vi "modbus_Unpuck.vi"(5 "Pair in":T1={"Давление заданное"=0.3, "Давление в системе"=99.99, "Расход заданый"=0.0, "Расход текущий"=0.0, "Объём заданный"=0.0, "Объём текущий"=0.0, "Старт давление"=FALSE, "Старт расход"=FALSE, "Сброс объёма"=FALSE, "plc_control"=FALSE, "lag_control"=FALSE, "mstop_control"=FALSE, "Давление"={"АЦП CH 0"=0.0, "АЦП CH 1"=0.0, "АЦП CH 2"=0.0, "АЦП CH 3"=0.0, "АЦП CH 4"=0.0, "АЦП CH 5"=0.0, "АЦП CH 6"=0.0, "АЦП CH 7"=0.0}, "Modbus"={"Массив чтения"=[], "Массив записи"=[]}} {"Давление"."АЦП CH 7" format="%.3f"; "Давление"."АЦП CH 6" format="%.3f"; "Давление"."АЦП CH 5" format="%.3f"; "Давление"."АЦП CH 4" format="%.3f"; "Давление"."АЦП CH 3" format="%.3f"; "Давление"."АЦП CH 2" format="%.3f"; "Давление"."АЦП CH 1" format="%.3f"; "Давление"."АЦП CH 0" format="%.3f"; "Объём текущий" min=0.0 max=9999.0 step=0.0001 format="%#_5f"; "Объём заданный" min=0.0 max=9999.0 step=0.0001 format="%#_5f"; "Расход текущий" format="%#_5f"; "Расход заданый" min=0.0 max=40.0 step=0.0001 format="%#_5f"; "Давление в системе" format="%.3f"; "Давление заданное" min=0.3 max=100.0 step=0.01 format="%#_5f"}, 6 "Параметры":T3, 7 "Port 2 in":T2={"Давление заданное"=0.3, "Давление MAX заданное"=100.0, "Давление в насосе"=0.0, "Давление в системе"=99.99, "Расход заданый"=0.0, "Расход текущий"=0.0, "Объём заданный"=0.0, "Объём текущий"=0.0, "Позиция насоса %"=0.0, "Ток двигателя"=0.0, "controlMsg"="", "Клапан k_sys"=FALSE, "Клапан k_res"=FALSE, "Клапан k_air"=FALSE, "Вверх"=FALSE, "Домой"=FALSE, "Вниз"=FALSE, "Старт расход"=FALSE, "Старт давление"=FALSE, "Сброс объёма"=FALSE, "Сброс давления Рсис"=FALSE, "Сброс давления Рнас"=FALSE, "Bits"={"plc_control"=FALSE, "lag_control"=FALSE, "mstop_control"=FALSE, "st_home"=FALSE, "error"=FALSE, "mstart"=FALSE, "pair"=FALSE, "startQ"=FALSE, "startP"=FALSE, "volume_Stop"=FALSE}} {"Ток двигателя" format="%#_5f"; "Расход текущий" format="%#_5f"; "Давление в системе" format="%.3f"; "Объём текущий" min=0.0 max=9999.0 step=0.0001 format="%#_5f"; "Объём заданный" min=0.0 max=9999.0 step=0.0001 format="%#_5f"; "Давление MAX заданное" min=0.0 max=100.0 step=0.01 format="%#_5f"; "Давление заданное" min=0.3 max=100.0 step=0.01 format="%#_5f"; "Расход заданый" min=0.0 max=40.0 step=0.0001 format="%#_5f"; "Давление в насосе" format="%.3f"; "Позиция насоса %" scale=0.0..100.0 scale format="%.2f"}, 8 "Error In":errorcluster, 10 "Modbus Read":u16[](array[numeric]), 11 "Port 1 in":T2={"Давление заданное"=0.3, "Давление MAX заданное"=100.0, "Давление в насосе"=0.0, "Давление в системе"=99.99, "Расход заданый"=0.0, "Расход текущий"=0.0, "Объём заданный"=0.0, "Объём текущий"=0.0, "Позиция насоса %"=0.0, "Ток двигателя"=0.0, "controlMsg"="", "Клапан k_sys"=FALSE, "Клапан k_res"=FALSE, "Клапан k_air"=FALSE, "Вверх"=FALSE, "Домой"=FALSE, "Вниз"=FALSE, "Старт расход"=FALSE, "Старт давление"=FALSE, "Сброс объёма"=FALSE, "Сброс давления Рсис"=FALSE, "Сброс давления Рнас"=FALSE, "Bits"={"plc_control"=FALSE, "lag_control"=FALSE, "mstop_control"=FALSE, "st_home"=FALSE, "error"=FALSE, "mstart"=FALSE, "pair"=FALSE, "startQ"=FALSE, "startP"=FALSE, "volume_Stop"=FALSE}} {"Ток двигателя" format="%#_5f"; "Расход текущий" format="%#_5f"; "Давление в системе" format="%.3f"; "Объём текущий" min=0.0 max=9999.0 step=0.0001 format="%#_5f"; "Объём заданный" min=0.0 max=9999.0 step=0.0001 format="%#_5f"; "Давление MAX заданное" min=0.0 max=100.0 step=0.01 format="%#_5f"; "Давление заданное" min=0.3 max=100.0 step=0.01 format="%#_5f"; "Расход заданый" min=0.0 max=40.0 step=0.0001 format="%#_5f"; "Давление в насосе" format="%.3f"; "Позиция насоса %" scale=0.0..100.0 scale format="%.2f"}) -> (0 "Error Out":errorcluster, 1 "Pair out":T1={"Давление заданное"=0.3, "Давление в системе"=99.99, "Расход заданый"=0.0, "Расход текущий"=0.0, "Объём заданный"=0.0, "Объём текущий"=0.0, "Старт давление"=FALSE, "Старт расход"=FALSE, "Сброс объёма"=FALSE, "plc_control"=FALSE, "lag_control"=FALSE, "mstop_control"=FALSE, "Давление"={"АЦП CH 0"=0.0, "АЦП CH 1"=0.0, "АЦП CH 2"=0.0, "АЦП CH 3"=0.0, "АЦП CH 4"=0.0, "АЦП CH 5"=0.0, "АЦП CH 6"=0.0, "АЦП CH 7"=0.0}, "Modbus"={"Массив чтения"=[], "Массив записи"=[]}} {"Давление"."АЦП CH 7" format="%.3f"; "Давление"."АЦП CH 6" format="%.3f"; "Давление"."АЦП CH 5" format="%.3f"; "Давление"."АЦП CH 4" format="%.3f"; "Давление"."АЦП CH 3" format="%.3f"; "Давление"."АЦП CH 2" format="%.3f"; "Давление"."АЦП CH 1" format="%.3f"; "Давление"."АЦП CH 0" format="%.3f"; "Объём текущий" min=0.0 max=9999.0 step=0.0001 format="%#_5f"; "Объём заданный" min=0.0 max=9999.0 step=0.0001 format="%#_5f"; "Расход текущий" format="%#_5f"; "Расход заданый" min=0.0 max=40.0 step=0.0001 format="%#_5f"; "Давление в системе" format="%.3f"; "Давление заданное" min=0.3 max=100.0 step=0.01 format="%#_5f"}, 2 "Port 2 out":T2={"Давление заданное"=0.3, "Давление MAX заданное"=100.0, "Давление в насосе"=0.0, "Давление в системе"=99.99, "Расход заданый"=0.0, "Расход текущий"=0.0, "Объём заданный"=0.0, "Объём текущий"=0.0, "Позиция насоса %"=0.0, "Ток двигателя"=0.0, "controlMsg"="", "Клапан k_sys"=FALSE, "Клапан k_res"=FALSE, "Клапан k_air"=FALSE, "Вверх"=FALSE, "Домой"=FALSE, "Вниз"=FALSE, "Старт расход"=FALSE, "Старт давление"=FALSE, "Сброс объёма"=FALSE, "Сброс давления Рсис"=FALSE, "Сброс давления Рнас"=FALSE, "Bits"={"plc_control"=FALSE, "lag_control"=FALSE, "mstop_control"=FALSE, "st_home"=FALSE, "error"=FALSE, "mstart"=FALSE, "pair"=FALSE, "startQ"=FALSE, "startP"=FALSE, "volume_Stop"=FALSE}} {"Ток двигателя" format="%#_5f"; "Расход текущий" format="%#_5f"; "Давление в системе" format="%.3f"; "Объём текущий" min=0.0 max=9999.0 step=0.0001 format="%#_5f"; "Объём заданный" min=0.0 max=9999.0 step=0.0001 format="%#_5f"; "Давление MAX заданное" min=0.0 max=100.0 step=0.01 format="%#_5f"; "Давление заданное" min=0.3 max=100.0 step=0.01 format="%#_5f"; "Расход заданый" min=0.0 max=40.0 step=0.0001 format="%#_5f"; "Давление в насосе" format="%.3f"; "Позиция насоса %" scale=0.0..100.0 scale format="%.2f"}, 3 "Port 1 out":T2={"Давление заданное"=0.3, "Давление MAX заданное"=100.0, "Давление в насосе"=0.0, "Давление в системе"=99.99, "Расход заданый"=0.0, "Расход текущий"=0.0, "Объём заданный"=0.0, "Объём текущий"=0.0, "Позиция насоса %"=0.0, "Ток двигателя"=0.0, "controlMsg"="", "Клапан k_sys"=FALSE, "Клапан k_res"=FALSE, "Клапан k_air"=FALSE, "Вверх"=FALSE, "Домой"=FALSE, "Вниз"=FALSE, "Старт расход"=FALSE, "Старт давление"=FALSE, "Сброс объёма"=FALSE, "Сброс давления Рсис"=FALSE, "Сброс давления Рнас"=FALSE, "Bits"={"plc_control"=FALSE, "lag_control"=FALSE, "mstop_control"=FALSE, "st_home"=FALSE, "error"=FALSE, "mstart"=FALSE, "pair"=FALSE, "startQ"=FALSE, "startP"=FALSE, "volume_Stop"=FALSE}} {"Ток двигателя" format="%#_5f"; "Расход текущий" format="%#_5f"; "Давление в системе" format="%.3f"; "Объём текущий" min=0.0 max=9999.0 step=0.0001 format="%#_5f"; "Объём заданный" min=0.0 max=9999.0 step=0.0001 format="%#_5f"; "Давление MAX заданное" min=0.0 max=100.0 step=0.01 format="%#_5f"; "Давление заданное" min=0.3 max=100.0 step=0.01 format="%#_5f"; "Расход заданый" min=0.0 max=40.0 step=0.0001 format="%#_5f"; "Давление в насосе" format="%.3f"; "Позиция насоса %" scale=0.0..100.0 scale format="%.2f"})   [LabVIEW 2023, in "pump_Lib.lvlib"]
uses:
  pump_Lib.lvlib
  TypeDef/pump_Type.ctl
  TypeDef/parametrs_Type.ctl
  TypeDef/pair_Type.ctl
  <vilib>/ptbypt/NI_PtbyPt.lvlib
panel:
  # "%"
  # "%"
  # "%"
  # "%"
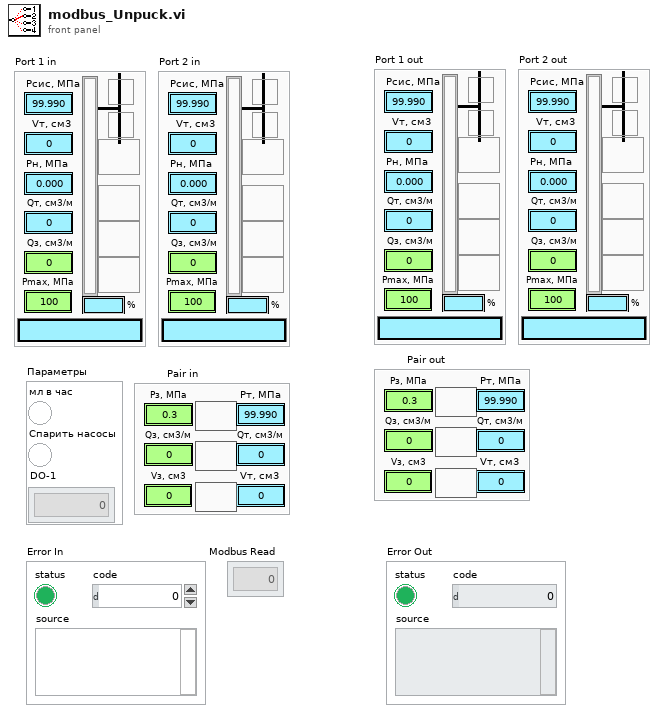
[diagram p1: front panel]
types:
  T1 = typedef "pump_Lib.lvlib/pair_Type.ctl" = cluster{"Давление заданное":dbl, "Давление в системе":dbl, "Расход заданый":dbl, "Расход текущий":dbl, "Объём заданный":dbl, "Объём текущий":dbl, "Старт давление":bool, "Старт расход":bool, "Сброс объёма":bool, "plc_control":bool, "lag_control":bool, "mstop_control":bool, "Давление":cluster{"АЦП CH 0":dbl, "АЦП CH 1":dbl, "АЦП CH 2":dbl, "АЦП CH 3":dbl, "АЦП CH 4":dbl, "АЦП CH 5":dbl, "АЦП CH 6":dbl, "АЦП CH 7":dbl}, "Modbus":cluster{"Массив чтения":u16[], "Массив записи":u16[]}}
  T2 = typedef "pump_Lib.lvlib/pump_Type.ctl" = cluster{"Давление заданное":dbl, "Давление MAX заданное":dbl, "Давление в насосе":dbl, "Давление в системе":dbl, "Расход заданый":dbl, "Расход текущий":dbl, "Объём заданный":dbl, "Объём текущий":dbl, "Позиция насоса %":dbl, "Ток двигателя":dbl, "controlMsg":string, "Клапан k_sys":bool, "Клапан k_res":bool, "Клапан k_air":bool, "Вверх":bool, "Домой":bool, "Вниз":bool, "Старт расход":bool, "Старт давление":bool, "Сброс объёма":bool, "Сброс давления Рсис":bool, "Сброс давления Рнас":bool, "Bits":cluster{"plc_control":bool, "lag_control":bool, "mstop_control":bool, "st_home":bool, "error":bool, "mstart":bool, "pair":bool, "startQ":bool, "startP":bool, "volume_Stop":bool}}
  T3 = typedef "pump_Lib.lvlib/parametrs_Type.ctl" = cluster{"мл в час":bool, "Спарить насосы":bool, "DO-1":u16[]}
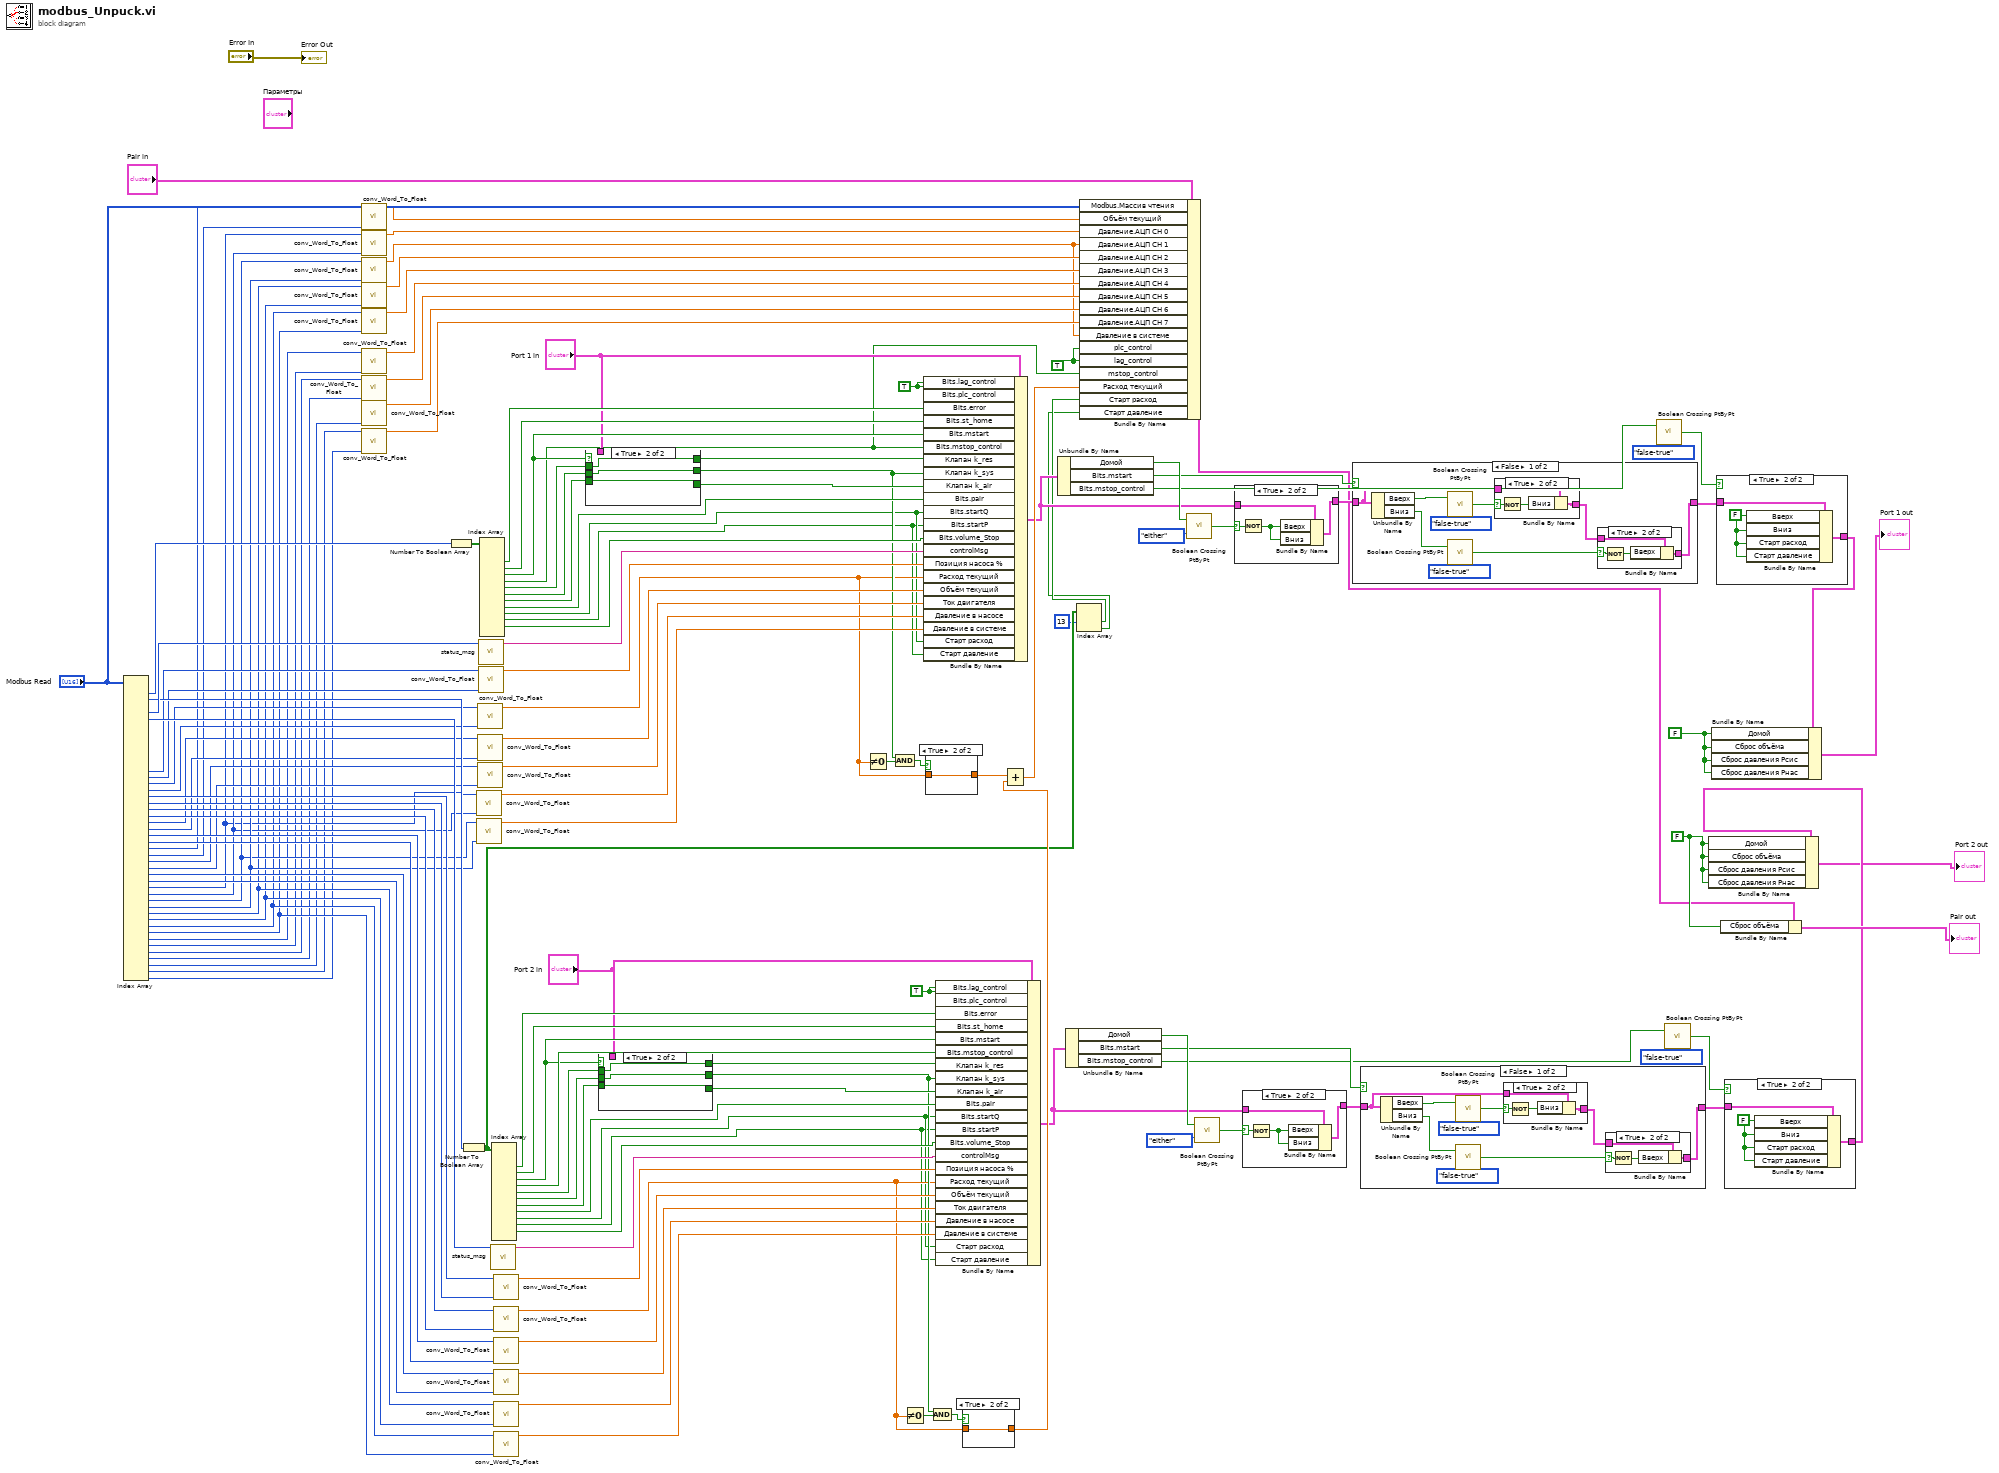
[diagram p0: block diagram]
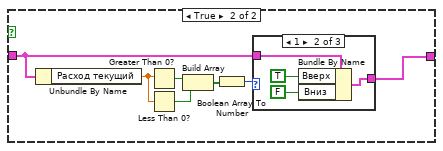
[diagram p5: hidden frame]
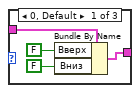
[diagram p6: hidden frame]
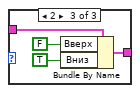
[diagram p7: hidden frame]
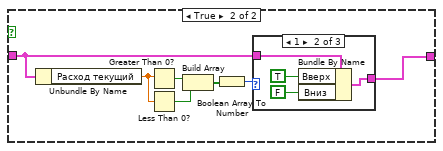
[diagram p12: hidden frame]
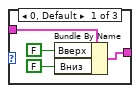
[diagram p13: hidden frame]
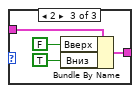
[diagram p14: hidden frame]
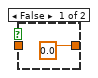
[diagram p16: hidden frame]
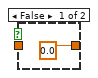
[diagram p17: hidden frame]
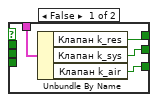
[diagram p18: hidden frame]
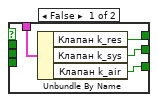
[diagram p19: hidden frame]
diagram:
  w15 = FALSE ("Домой")
  w16 = FALSE ("Домой")
  w40 = TRUE ("plc_control")
  w46 = TRUE ("plc_control")
  w47 = TRUE ("plc_control")
  n1 = Index Array(array="Modbus Read") -> (element #1=w136:u16, element #2=w108:u16, element #4=w134:u16, element #5=w107:u16, element #13=w106:u16, element #14=w105:u16, element #15=w104:u16, element #16=w103:u16, element #17=w100:u16, element #18=w99:u16, element #19=w98:u16, element #20=w97:u16, element #21=w95:u16, element #22=w94:u16, element #23=w92:u16, element #24=w91:u16, element #25=w88:u16, element #26=w87:u16, element #27=w85:u16, element #28=w84:u16, element #29=w83:u16, element #30=w82:u16, element #31=w64:u16, element #32=w65:u16, element #33=w66:u16, element #34=w67:u16, element #35=w63:u16, element #36=w62:u16, element #37=w61:u16, element #38=w60:u16, element #39=w59:u16, element #40=w58:u16, element #41=w57:u16, element #42=w56:u16, element #43=w55:u16, element #44=w54:u16, element #45=w53:u16)  [unwired: 45 in, 8 out]
  n2 = call "conv_Word_To_Float.vi"("second_Word"=w87, "first_Word"=w88) -> ("output_Float"=w80:sgl)  [unwired: 9 in]
  n3 = call "conv_Word_To_Float.vi"("second_Word"=w65, "first_Word"=w64) -> ("output_Float"=w77:sgl)  [unwired: 9 in]
  n4 = call "conv_Word_To_Float.vi"("second_Word"=w67, "first_Word"=w66) -> ("output_Float"=w68:sgl)  [unwired: 9 in]
  n5 = call "conv_Word_To_Float.vi"("second_Word"=w62, "first_Word"=w63) -> ("output_Float"=w76:sgl)  [unwired: 9 in]
  n6 = call "conv_Word_To_Float.vi"("second_Word"=w60, "first_Word"=w61) -> ("output_Float"=w75:sgl)  [unwired: 9 in]
  n7 = call "conv_Word_To_Float.vi"("second_Word"=w58, "first_Word"=w59) -> ("output_Float"=w74:sgl)  [unwired: 9 in]
  n8 = call "conv_Word_To_Float.vi"("second_Word"=w56, "first_Word"=w57) -> ("output_Float"=w73:sgl)  [unwired: 9 in]
  n9 = call "conv_Word_To_Float.vi"("second_Word"=w55) -> ("output_Float"=w72:sgl)  [unwired: 10 in]
  n10 = call "conv_Word_To_Float.vi"("second_Word"=w53, "first_Word"=w54) -> ("output_Float"=w71:sgl)  [unwired: 9 in]
  n11 = Number To Boolean Array(number=w136) -> (Boolean array=w135:bool[])
  n12 = Number To Boolean Array(number=w108) -> (Boolean array=w8:bool[])
  n13 = call "conv_Word_To_Float.vi"("second_Word"=w65, "first_Word"=w64) -> ("output_Float"=w79:sgl)  [unwired: 9 in]
  n14 = call "conv_Word_To_Float.vi"("second_Word"=w67, "first_Word"=w66) -> ("output_Float"=w78:sgl)  [unwired: 9 in]
  n15 = call "conv_Word_To_Float.vi"("second_Word"=w103, "first_Word"=w104) -> ("output_Float"=w48:sgl)  [unwired: 9 in]
  n16 = call "conv_Word_To_Float.vi"("second_Word"=w94, "first_Word"=w95) -> ("output_Float"=w96:sgl)  [unwired: 9 in]
  n17 = call "conv_Word_To_Float.vi"("second_Word"=w84, "first_Word"=w85) -> ("output_Float"=w86:sgl)  [unwired: 9 in]
  n18 = call "status_msg.vi"("status_Word"=w134) -> ("controlMsg"=w122:string)  [unwired: 10 in]
  n19 = call "conv_Word_To_Float.vi"("second_Word"=w105, "first_Word"=w106) -> ("output_Float"=w102:sgl)  [unwired: 9 in]
  n20 = Index Array(array=w135) -> (element #2=w133:bool, element #3=w132:bool, element #4=w129:bool, element #5=w41:bool, element #6=w128:bool, element #7=w127:bool, element #8=w126:bool, element #9=w124:bool, element #10=w4:bool, element #11=w3:bool, element #12=w123:bool)  [unwired: 13 in, 2 out]
  n21 = call "status_msg.vi"("status_Word"=w107) -> ("controlMsg"=w110:string)  [unwired: 10 in]
  n22 = Index Array(array=w8) -> (element #2=w121:bool, element #3=w120:bool, element #4=w116:bool, element #5=w119:bool, element #6=w115:bool, element #7=w114:bool, element #8=w113:bool, element #9=w112:bool, element #10=w2:bool, element #11=w1:bool, element #12=w111:bool)  [unwired: 13 in, 2 out]
  n23 = call "conv_Word_To_Float.vi"("second_Word"=w99, "first_Word"=w100) -> ("output_Float"=w101:sgl)  [unwired: 9 in]
  n24 = call "conv_Word_To_Float.vi"("second_Word"=w97, "first_Word"=w98) -> ("output_Float"=w42:sgl)  [unwired: 9 in]
  n25 = call "conv_Word_To_Float.vi"("second_Word"=w91, "first_Word"=w92) -> ("output_Float"=w93:sgl)  [unwired: 9 in]
  n26 = call "conv_Word_To_Float.vi"("second_Word"=w82, "first_Word"=w83) -> ("output_Float"=w81:sgl)  [unwired: 9 in]
  n27 = call "conv_Word_To_Float.vi"("second_Word"=w62, "first_Word"=w63) -> ("output_Float"=w70:sgl)  [unwired: 9 in]
  n28 = call "conv_Word_To_Float.vi"("second_Word"=w60, "first_Word"=w61) -> ("output_Float"=w69:sgl)  [unwired: 9 in]
  n29 = case shown="True" w129 {
    tunnel: [w139 w143] -> w131
    tunnel: [w138 w142] -> w50
    tunnel: [w137 w141] -> w130
    tunnel: w128 -> [_ w143]
    tunnel: w127 -> [_ w142]
    tunnel: w126 -> [_ w141]
    tunnel: "Port 1 in" -> [w140 _]
    frame False {
      n30 = Unbundle By Name(w140) -> ("Клапан k_res"=w139:bool, "Клапан k_sys"=w138:bool, "Клапан k_air"=w137:bool)
    }
    frame True {
    }
  }
  n31 = case shown="True" w116 {
    tunnel: [w146 w150] -> w118
    tunnel: [w145 w149] -> w43
    tunnel: [w144 w148] -> w117
    tunnel: w115 -> [_ w150]
    tunnel: w114 -> [_ w149]
    tunnel: w113 -> [_ w148]
    tunnel: "Port 2 in" -> [w147 _]
    frame False {
      n32 = Unbundle By Name(w147) -> ("Клапан k_res"=w146:bool, "Клапан k_sys"=w145:bool, "Клапан k_air"=w144:bool)
    }
    frame True {
    }
  }
  n33 = Not Equal To 0?(x=w48) -> (x != 0?=w51:bool)
  n34 = And(x=w50, y=w51) -> (x .and. y?=w49:bool)
  n35 = Not Equal To 0?(x=w42) -> (x != 0?=w45:bool)
  n36 = Bundle By Name(cluster="Port 1 in", "Bits.lag_control"=w47, "Bits.plc_control"=w47, "Bits.error"=w133, "Bits.st_home"=w132, "Bits.mstart"=w129, "Bits.mstop_control"=w41, "Клапан k_res"=w131, "Клапан k_sys"=w50, "Клапан k_air"=w130, "Bits.pair"=w124, "Bits.startQ"=w4, "Bits.startP"=w3, "Bits.volume_Stop"=w123, "controlMsg"=w122, "Позиция насоса %"=w102, "Расход текущий"=w48, "Объём текущий"=w96, "Ток двигателя"=w86, "Давление в насосе"=w79, "Давление в системе"=w78, "Старт расход"=w4, "Старт давление"=w3) -> (w33:T2)
  n37 = case shown="True" w49 {
    tunnel: w48 -> [_ w152]
    tunnel: [0.0 ("SR") w152] -> w39
    frame False {
    }
    frame True {
    }
  }
  n38 = And(x=w43, y=w45) -> (x .and. y?=w44:bool)
  n39 = Bundle By Name(cluster="Port 2 in", "Bits.lag_control"=w46, "Bits.plc_control"=w46, "Bits.error"=w121, "Bits.st_home"=w120, "Bits.mstart"=w116, "Bits.mstop_control"=w119, "Клапан k_res"=w118, "Клапан k_sys"=w43, "Клапан k_air"=w117, "Bits.pair"=w112, "Bits.startQ"=w2, "Bits.startP"=w1, "Bits.volume_Stop"=w111, "controlMsg"=w110, "Позиция насоса %"=w101, "Расход текущий"=w42, "Объём текущий"=w93, "Ток двигателя"=w81, "Давление в насосе"=w70, "Давление в системе"=w69, "Старт расход"=w2, "Старт давление"=w1) -> (w17:T2)
  n40 = case shown="True" w44 {
    tunnel: w42 -> [_ w154]
    tunnel: [0.0 ("SR") w154] -> w38
    frame False {
    }
    frame True {
    }
  }
  n41 = Add(x=w39, y=w38) -> (x+y=w37:dbl)
  n42 = Unbundle By Name(w33) -> ("Домой"=w34:bool, "Bits.mstart"=w31:bool, "Bits.mstop_control"=w28:bool)
  n43 = Unbundle By Name(w17) -> ("Домой"=w24:bool, "Bits.mstart"=w22:bool, "Bits.mstop_control"=w19:bool)
  n44 = Index Array(array=w8, index #1=13 ("index")) -> (element #1=w6:bool, element #2=w5:bool)  [unwired: 1 in]
  n45 = Bundle By Name(cluster="Pair in", "Modbus.Массив чтения"="Modbus Read", "Объём текущий"=w80, "Давление.АЦП CH 0"=w77, "Давление.АЦП CH 1"=w68, "Давление.АЦП CH 2"=w76, "Давление.АЦП CH 3"=w75, "Давление.АЦП CH 4"=w74, "Давление.АЦП CH 5"=w73, "Давление.АЦП CH 6"=w72, "Давление.АЦП CH 7"=w71, "Давление в системе"=w68, "plc_control"=w40, "lag_control"=w40, "mstop_control"=w41, "Расход текущий"=w37, "Старт расход"=w6, "Старт давление"=w5) -> (w12:T1)
  n46 = call <vilib>:"Boolean Crossing PtByPt.vi"("direction"=enum16{"either", "false-true", "true-false"}."either", "input"=w34) -> ("crossing"=w35:bool)  [unwired: 1 in]
  n47 = call <vilib>:"Boolean Crossing PtByPt.vi"("direction"=enum16{"either", "false-true", "true-false"}."either", "input"=w24) -> ("crossing"=w25:bool)  [unwired: 1 in]
  n48 = case shown="True" w35 {
    selector: w35 -> [_ w156]
    tunnel: w33 -> [w155 w159]
    tunnel: [w155 w157] -> w32
    frame False {
    }
    frame True {
      n49 = Not(x=w156) -> (.not. x?=w158:bool)
      n50 = Bundle By Name(cluster=w159, "Вверх"=w158, "Вниз"=w158) -> (w157:T2)
    }
  }
  n51 = case shown="True" w25 {
    selector: w25 -> [_ w161]
    tunnel: w17 -> [w160 w164]
    tunnel: [w160 w162] -> w23
    frame False {
    }
    frame True {
      n52 = Not(x=w161) -> (.not. x?=w163:bool)
      n53 = Bundle By Name(cluster=w164, "Вверх"=w163, "Вниз"=w163) -> (w162:T2)
    }
  }
  n54 = case shown="False" w31 {
    tunnel: w32 -> [w171 w190]
    tunnel: [w165 w184] -> w27
    frame False {
      n55 = Unbundle By Name(w171) -> ("Вверх"=w169:bool, "Вниз"=w168:bool)
      n56 = call <vilib>:"Boolean Crossing PtByPt.vi"("direction"=enum16{"either", "false-true", "true-false"}."false-true", "input"=w169) -> ("crossing"=w170:bool)  [unwired: 1 in]
      n57 = call <vilib>:"Boolean Crossing PtByPt.vi"("direction"=enum16{"either", "false-true", "true-false"}."false-true", "input"=w168) -> ("crossing"=w166:bool)  [unwired: 1 in]
      n58 = case shown="True" w170 {
        selector: w170 -> [_ w182]
        tunnel: w171 -> [w179 w181]
        tunnel: [w179 w180] -> w167
        frame False {
        }
        frame True {
          n59 = Not(x=w182) -> (.not. x?=w183:bool)
          n60 = Bundle By Name(cluster=w181, "Вниз"=w183) -> (w180:T2)
        }
      }
      n61 = case shown="True" w166 {
        selector: w166 -> [_ w177]
        tunnel: w167 -> [w174 w176]
        tunnel: [w174 w175] -> w165
        frame False {
        }
        frame True {
          n62 = Not(x=w177) -> (.not. x?=w178:bool)
          n63 = Bundle By Name(cluster=w176, "Вверх"=w178) -> (w175:T2)
        }
      }
    }
    frame True {
      n64 = Unbundle By Name(w190) -> ("Расход текущий"=w189:dbl)
      n65 = Greater Than 0?(x=w189) -> (x > 0?=w188:bool)
      n66 = Less Than 0?(x=w189) -> (x < 0?=w187:bool)
      n67 = Build Array(w188, w187) -> (w186:bool[])
      n68 = Boolean Array To Number(Boolean array=w186) -> (number=w185:u32)
      n69 = case shown="1" w185 {
        tunnel: w190 -> [w192 w196 w202]
        tunnel: [w191 w195 w199] -> w184
        frame 0, Default {
          n70 = Bundle By Name(cluster=w192, "Вверх"=FALSE, "Вниз"=FALSE) -> (w191:T2)
        }
        frame 1 {
          n71 = Bundle By Name(cluster=w196, "Вверх"=TRUE, "Вниз"=FALSE) -> (w195:T2)
        }
        frame 2 {
          n72 = Bundle By Name(cluster=w202, "Вверх"=FALSE, "Вниз"=TRUE) -> (w199:T2)
        }
      }
    }
  }
  n73 = case shown="False" w22 {
    tunnel: w23 -> [w209 w228]
    tunnel: [w203 w222] -> w18
    frame False {
      n74 = Unbundle By Name(w209) -> ("Вверх"=w207:bool, "Вниз"=w206:bool)
      n75 = call <vilib>:"Boolean Crossing PtByPt.vi"("direction"=enum16{"either", "false-true", "true-false"}."false-true", "input"=w207) -> ("crossing"=w208:bool)  [unwired: 1 in]
      n76 = call <vilib>:"Boolean Crossing PtByPt.vi"("direction"=enum16{"either", "false-true", "true-false"}."false-true", "input"=w206) -> ("crossing"=w204:bool)  [unwired: 1 in]
      n77 = case shown="True" w208 {
        selector: w208 -> [_ w220]
        tunnel: w209 -> [w217 w219]
        tunnel: [w217 w218] -> w205
        frame False {
        }
        frame True {
          n78 = Not(x=w220) -> (.not. x?=w221:bool)
          n79 = Bundle By Name(cluster=w219, "Вниз"=w221) -> (w218:T2)
        }
      }
      n80 = case shown="True" w204 {
        selector: w204 -> [_ w215]
        tunnel: w205 -> [w212 w214]
        tunnel: [w212 w213] -> w203
        frame False {
        }
        frame True {
          n81 = Not(x=w215) -> (.not. x?=w216:bool)
          n82 = Bundle By Name(cluster=w214, "Вверх"=w216) -> (w213:T2)
        }
      }
    }
    frame True {
      n83 = Unbundle By Name(w228) -> ("Расход текущий"=w227:dbl)
      n84 = Greater Than 0?(x=w227) -> (x > 0?=w226:bool)
      n85 = Less Than 0?(x=w227) -> (x < 0?=w225:bool)
      n86 = Build Array(w226, w225) -> (w224:bool[])
      n87 = Boolean Array To Number(Boolean array=w224) -> (number=w223:u32)
      n88 = case shown="1" w223 {
        tunnel: w228 -> [w230 w234 w240]
        tunnel: [w229 w233 w237] -> w222
        frame 0, Default {
          n89 = Bundle By Name(cluster=w230, "Вверх"=FALSE, "Вниз"=FALSE) -> (w229:T2)
        }
        frame 1 {
          n90 = Bundle By Name(cluster=w234, "Вверх"=TRUE, "Вниз"=FALSE) -> (w233:T2)
        }
        frame 2 {
          n91 = Bundle By Name(cluster=w240, "Вверх"=FALSE, "Вниз"=TRUE) -> (w237:T2)
        }
      }
    }
  }
  n92 = call <vilib>:"Boolean Crossing PtByPt.vi"("direction"=enum16{"either", "false-true", "true-false"}."false-true", "input"=w28) -> ("crossing"=w29:bool)  [unwired: 1 in]
  n93 = call <vilib>:"Boolean Crossing PtByPt.vi"("direction"=enum16{"either", "false-true", "true-false"}."false-true", "input"=w19) -> ("crossing"=w20:bool)  [unwired: 1 in]
  n94 = case shown="True" w29 {
    tunnel: w27 -> [w241 w244]
    tunnel: [w241 w243] -> w14
    frame False {
    }
    frame True {
      w242 = FALSE
      n95 = Bundle By Name(cluster=w244, "Вверх"=w242, "Вниз"=w242, "Старт расход"=w242, "Старт давление"=w242) -> (w243:T2)
    }
  }
  n96 = Bundle By Name(cluster=w14, "Домой"=w16, "Сброс объёма"=w16, "Сброс давления Рсис"=w16, "Сброс давления Рнас"=w16) -> (→"Port 1 out":T2)
  n97 = Bundle By Name(cluster=w12, "Сброс объёма"=w15) -> (→"Pair out":T1)
  n98 = case shown="True" w20 {
    tunnel: w18 -> [w245 w248]
    tunnel: [w245 w247] -> w10
    frame False {
    }
    frame True {
      w246 = FALSE
      n99 = Bundle By Name(cluster=w248, "Вверх"=w246, "Вниз"=w246, "Старт расход"=w246, "Старт давление"=w246) -> (w247:T2)
    }
  }
  n100 = Bundle By Name(cluster=w10, "Домой"=w15, "Сброс объёма"=w15, "Сброс давления Рсис"=w15, "Сброс давления Рнас"=w15) -> (→"Port 2 out":T2)
  "Error Out" <- "Error In"
